vi "VariantToPlainText.vi"(7 "use system decimal point (T)":bool=TRUE, 11 "Variant-formatted Value":variant) -> (3 "String-formatted Value":string)   [LabVIEW 2013, in "Serializer.PlainText.lvclass"]
uses:
  Serializer.PlainText.lvclass
  <vilib>/Utility/VariantDataType/VariantType.lvlib
  <vilib>/LabVIEW Open Source Project/Data Manipulation/TypeDescriptor/OpenDescriptor.lvlib
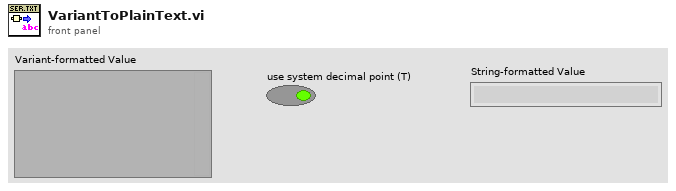
[diagram p1: front panel]
types:
  T1 = typedef "VariantType.lvlib/Type.ctl" = enum8{"Invalid Type", "Void", "I8", "I16", "I32", "I64", "U8", "U16", "U32", "U64", "Single Float", "Double Float", "Extended Float", "Single Complex", "Double Complex", "Extended Complex", "Enum U8", "Enum U16", "Enum U32", "Enum U64", "Single Float With Unit", "Double Float With Unit", "Extended Float With Unit", "Single Complex with Unit", "Double Complex with Unit", "Extended Complex with Unit", "Boolean", "String", "Path", "Picture", "Tag", "Array", "Cluster", "Variant", "LV Variant", "Waveform", "Timestamp", "Digital Waveform", "Digital Data", "ExpressData", "Refnum", "External Data", "VI", "Poly VI", "LabVIEW Class Instance", "Fixed Point"}
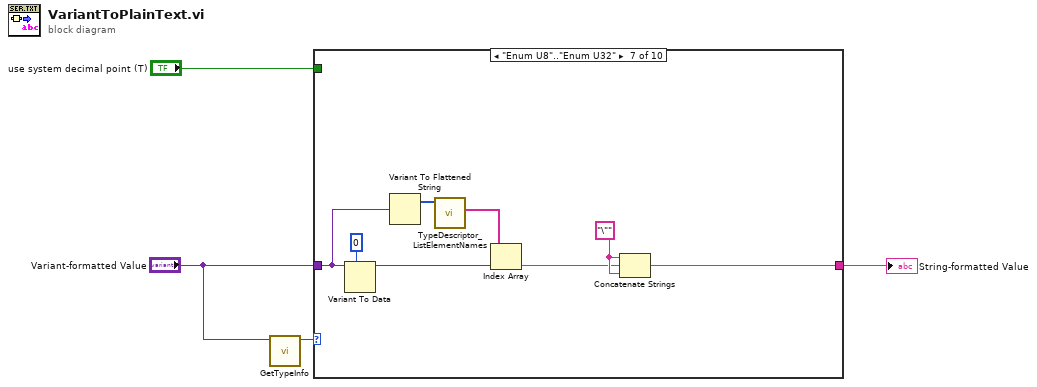
[diagram p0: block diagram]
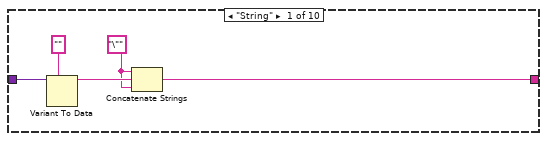
[diagram p2: hidden frame]
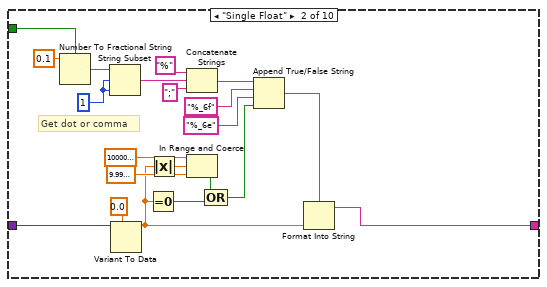
[diagram p3: hidden frame]
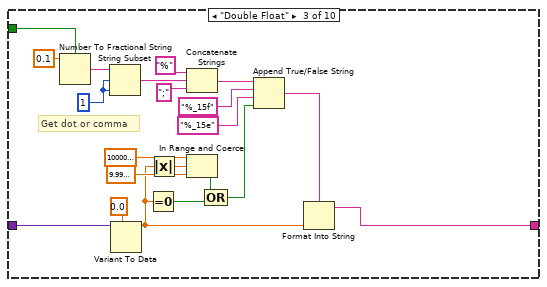
[diagram p4: hidden frame]
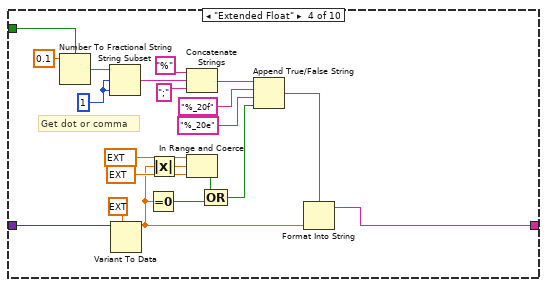
[diagram p5: hidden frame]
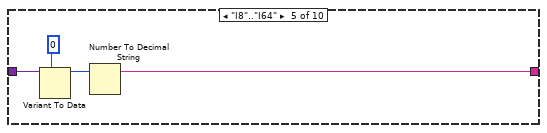
[diagram p6: hidden frame]
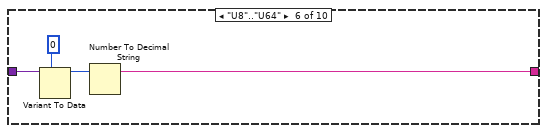
[diagram p7: hidden frame]
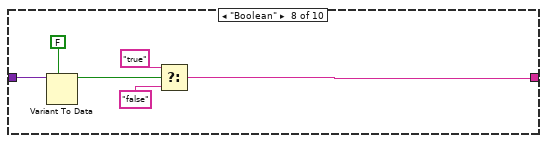
[diagram p8: hidden frame]
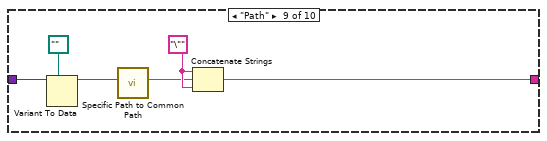
[diagram p9: hidden frame]
diagram:
  n1 = call <vilib>:"GetTypeInfo.vi"("Variant"="Variant-formatted Value") -> ("Type Enum"=w4:T1)  [unwired: 6 in, 4 out]
  n2 = case shown="\"Enum U8\"..\"Enum U32\"" w4 {
    tunnel: "Variant-formatted Value" -> [w9 w23 w44 w65 w74 w78 w87 w94 w100 _]
    tunnel: [w6 w10 w31 w52 w73 w77 w81 w91 w97 _] -> w1
    tunnel: "use system decimal point (T)" -> [_ w21 w42 w63 _ _ _ _ _ _]
    frame "String" {
      w5 = "\"" ("Format String")
      n3 = Variant To Data(type="" ("Format String"), Variant=w9) -> (data=w7:string)  [unwired: 1 in, 1 out]
      n4 = Concatenate Strings(w5, w7, w5) -> (w6:string)
    }
    frame "Single Float" {
      w19 = 1 ("length (rest)")
      # "Get dot or comma"
      n5 = Number To Fractional String(use system decimal point (T)=w21, number=0.1) -> (F-format string=w20:string)  [unwired: 2 in]
      n6 = String Subset(string=w20, offset (0)=w19, length (rest)=w19) -> (substring=w18:string)
      n7 = Variant To Data(type=sgl 0.0, Variant=w23) -> (data=w26:sgl)  [unwired: 1 in, 1 out]
      n8 = Equal To 0?(x=w26) -> (x = 0?=w25:bool)
      n9 = Absolute Value(x=w26) -> (abs(x)=w27:sgl)
      n10 = Concatenate Strings("%" ("format string"), w18, ";" ("format string")) -> (w15:string)
      n11 = In Range and Coerce(upper limit=sgl 1000000.0, x=w27, lower limit=sgl 0.0001 ("upper limit")) -> (In Range?=w24:bool)  [unwired: 1 out]
      n12 = Compound Arithmetic op=OR(w24, w25) -> (w12:bool)
      n13 = Append True/False String(1:w12, 2:"%_6e" ("format string"), 3:"%_6f" ("format string"), 4:w15) -> (0:w11:string)
      n14 = Format Into String(format string=w11, w26) -> (resulting string=w10:string)  [unwired: 2 in, 1 out]
    }
    frame "Double Float" {
      w40 = 1 ("length (rest)")
      # "Get dot or comma"
      n15 = Number To Fractional String(use system decimal point (T)=w42, number=0.1) -> (F-format string=w41:string)  [unwired: 2 in]
      n16 = String Subset(string=w41, offset (0)=w40, length (rest)=w40) -> (substring=w39:string)
      n17 = Variant To Data(type=0.0, Variant=w44) -> (data=w47:dbl)  [unwired: 1 in, 1 out]
      n18 = Equal To 0?(x=w47) -> (x = 0?=w46:bool)
      n19 = Absolute Value(x=w47) -> (abs(x)=w48:dbl)
      n20 = Concatenate Strings("%" ("format string"), w39, ";" ("format string")) -> (w36:string)
      n21 = In Range and Coerce(upper limit=1000000.0, x=w48, lower limit=9.999999747378752e-05 ("upper limit")) -> (In Range?=w45:bool)  [unwired: 1 out]
      n22 = Compound Arithmetic op=OR(w45, w46) -> (w33:bool)
      n23 = Append True/False String(1:w33, 2:"%_15e" ("format string"), 3:"%_15f" ("format string"), 4:w36) -> (0:w32:string)
      n24 = Format Into String(format string=w32, w47) -> (resulting string=w31:string)  [unwired: 2 in, 1 out]
    }
    frame "Extended Float" {
      w61 = 1 ("length (rest)")
      # "Get dot or comma"
      n25 = Number To Fractional String(use system decimal point (T)=w63, number=0.1) -> (F-format string=w62:string)  [unwired: 2 in]
      n26 = String Subset(string=w62, offset (0)=w61, length (rest)=w61) -> (substring=w60:string)
      n27 = Variant To Data(type=ext 0.0, Variant=w65) -> (data=w68:ext)  [unwired: 1 in, 1 out]
      n28 = Equal To 0?(x=w68) -> (x = 0?=w67:bool)
      n29 = Absolute Value(x=w68) -> (abs(x)=w69:ext)
      n30 = Concatenate Strings("%" ("format string"), w60, ";" ("format string")) -> (w57:string)
      n31 = In Range and Coerce(upper limit=ext 1000000.0, x=w69, lower limit=ext 9.999999747378752e-05 ("upper limit")) -> (In Range?=w66:bool)  [unwired: 1 out]
      n32 = Compound Arithmetic op=OR(w66, w67) -> (w54:bool)
      n33 = Append True/False String(1:w54, 2:"%_20e" ("format string"), 3:"%_20f" ("format string"), 4:w57) -> (0:w53:string)
      n34 = Format Into String(format string=w53, w68) -> (resulting string=w52:string)  [unwired: 2 in, 1 out]
    }
    frame "I8".."I64" {
      n35 = Variant To Data(type=i64 0, Variant=w74) -> (data=w75:i64)  [unwired: 1 in, 1 out]
      n36 = Number To Decimal String(number=w75) -> (decimal integer string=w73:string)  [unwired: 1 in]
    }
    frame "U8".."U64" {
      n37 = Variant To Data(type=u64 0, Variant=w78) -> (data=w79:u64)  [unwired: 1 in, 1 out]
      n38 = Number To Decimal String(number=w79) -> (decimal integer string=w77:string)  [unwired: 1 in]
    }
    frame "Enum U8".."Enum U32" {
      w83 = "\"" ("Format String")
      n39 = Variant To Data(type=0, Variant=w87) -> (data=w84:i32)  [unwired: 1 in, 1 out]
      n40 = Variant To Flattened String(Variant=w87) -> (1:w86:i16[])  [unwired: 1 out]
      n41 = call <vilib>:"TypeDescriptor_ListElementNames.vi"("type descriptor"=w86) -> ("element names"=w85:string[])  [unwired: 8 in, 2 out]
      n42 = Index Array(array=w85, index=w84) -> (element=w82:string)
      n43 = Concatenate Strings(w83, w82, w83) -> (w81:string)
    }
    frame "Boolean" {
      n44 = Variant To Data(type=FALSE, Variant=w94) -> (data=w92:bool)  [unwired: 1 in, 1 out]
      n45 = Select(t="true", s=w92, f="false") -> (s? t:f=w91:string)
    }
    frame "Path" {
      w98 = "\"" ("Format String")
      n46 = Variant To Data(type=path "" ("Format String"), Variant=w100) -> (data=w96:path)  [unwired: 1 in, 1 out]
      n47 = call "Specific Path to Common Path.vi"("specific path"=w96) -> ("common path"=w95:string)  [unwired: 10 in]
      n48 = Concatenate Strings(w98, w95, w98) -> (w97:string)
    }
    frame Default {
    }
  }
  "String-formatted Value" <- w1
